vi "Get Connections with Session.vi"(0 "Keysight_34401A-DMM in":refnum<class "Keysight_34401A-DMM.lvclass">, 5 "pin or relay names":string[](array[string]), 11 "error in (no error)":errorcluster, 12 "site":i32, 13 "pin type":T1) -> (4 "Keysight_34401A-DMM out":refnum<class "Keysight_34401A-DMM.lvclass">, 6 "connections":T2[](array[typedef]), 15 "error out":errorcluster)   [LabVIEW 2020, in "Abstract_Instrument.lvlib" / "Keysight_34401A-DMM.lvclass"]
uses:
  Keysight_34401A-DMM.lvclass
  TypeDef/Connection with Session.ctl
  <vilib>/MeasurementLink/MeasurementLink Session Management V1/Session Reservation/Connection.ctl
  C:/Program Files/National Instruments/LabVIEW 2020/vi.lib/MeasurementLink/MeasurementLink Instrument/ISession Factory/ISession Factory.lvclass
  <vilib>/MeasurementLink/MeasurementLink Session Management V1/Session Reservation/Pin Type.ctl
  3de7b559-e2a1-4487-9d2e-597741313616.vi
  <vilib>/MeasurementLink/MeasurementLink Session Management V1/Session Reservation/Get Connections Impl.vi
  <vilib>/MeasurementLink/MeasurementLink Session Management V1/Session Reservation/Session Reservation.lvclass
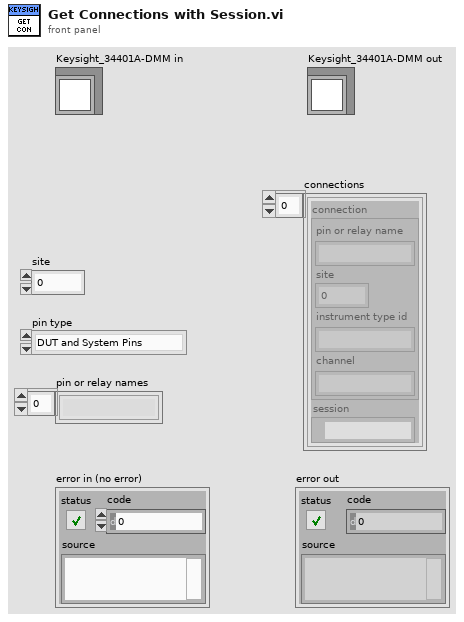
[diagram p1: front panel]
types:
  T1 = typedef "MeasurementLink Session Management V1.lvlib/Session Reservation.lvclass/Pin Type.ctl" = enum16{"DUT and System Pins", "System Pins"}
  T2 = typedef "Abstract_Instrument.lvlib/Keysight_34401A-DMM.lvclass/Connection with Session.ctl" = cluster{"connection":T3, "session":refnum<visa-resource-name>}
  T3 = typedef "MeasurementLink Session Management V1.lvlib/Session Reservation.lvclass/Connection.ctl" = cluster{"pin or relay name":string, "site":i32, "instrument type id":string, "channel":string}
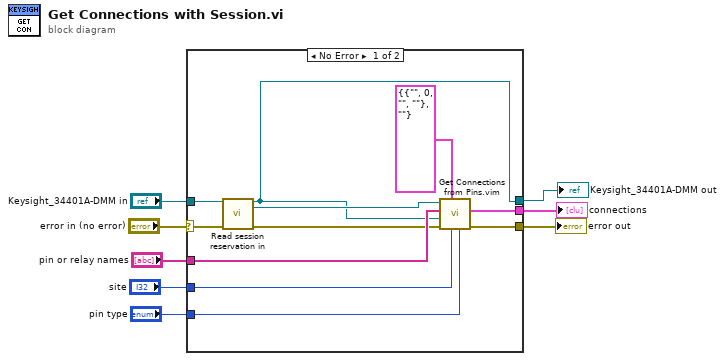
[diagram p0: block diagram]
diagram:
  n1 = case shown="No Error" "error in (no error)" {
    selector: "error in (no error)" -> [w13 w21]
    tunnel: [w19 _] -> w8
    tunnel: "pin or relay names" -> [w17 _]
    tunnel: [w16 w21] -> w6
    tunnel: "Keysight_34401A-DMM in" -> [w12 w20]
    tunnel: [w11 w20] -> w3
    tunnel: "site" -> [w10 _]
    tunnel: "pin type" -> [w9 _]
    frame No Error {
      n2 = call-dynamic "Read session reservation in.vi"("AbstractDMM in"=w12, "error in (no error)"=w13) -> ("AbstractDMM out"=w11:refnum<class "Keysight_34401A-DMM.lvclass">, "MeasurementLink Session Management V1.lvlib:Session Reservation.lvclass"=w14:refnum<class "Session Reservation.lvclass">, "error out"=w15:errorcluster)  [unwired: 11 in]
      n3 = call "Get Connections from Pins.vim"("pin type"=w9, "site"=w10, "connection type"=T2 {"connection"={"pin or relay name"="", "site"=0, "instrument type id"="", "channel"=""}, "session"=""}, "error in"=w15, "session factory"=w11, "pin or relay names"=w17, "session reservation in"=w14) -> ("error out"=w16:errorcluster, "connections"=w19:T2[])  [unwired: 2 in, 1 out]
    }
    frame Error {
    }
  }
  "connections" <- w8
  "error out" <- w6
  "Keysight_34401A-DMM out" <- w3
